vi "IsSearchGoalNode.vi"(8 "error in (no error)":errorcluster, 10 "PossibleSearchGoal in":refnum<data-value>, 11 "Tree in":refnum<class "Tree.lvclass">) -> (0 "error out":errorcluster, 1 "IsNode":bool, 2 "PossibleSearchGoal out":refnum<data-value>, 3 "Tree out":refnum<class "Tree.lvclass">)   [LabVIEW 2013, in "Tree.lvclass"]
doc: "Abstract method. Override this VI to implement a search of a tree. This VI is responsible for determining when we have found the node we are searching for."
uses:
  Tree.lvclass
  TreeNode/TreeNode.lvclass
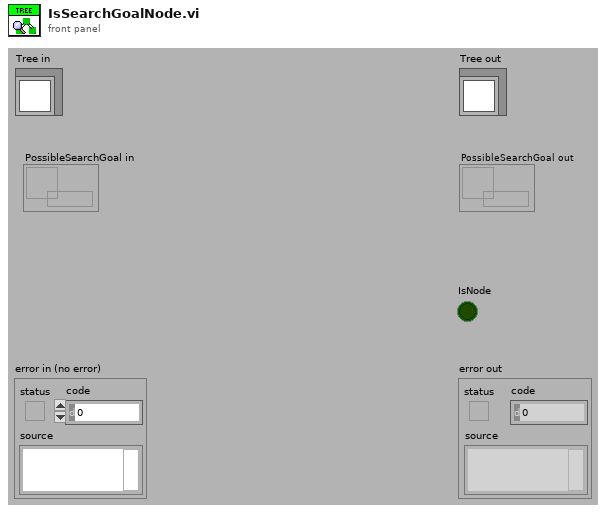
[diagram p1: front panel]
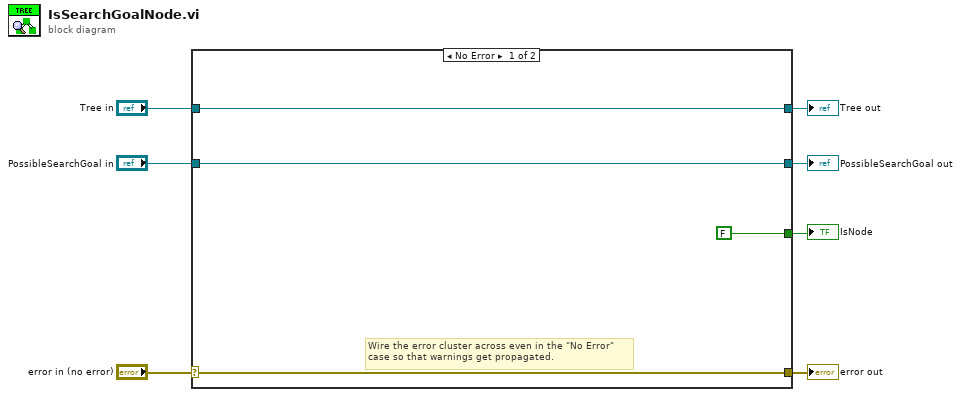
[diagram p0: block diagram]
diagram:
  n1 = case shown="No Error" "error in (no error)" {
    selector: "error in (no error)" -> [w10 w14]
    tunnel: [w10 w14] -> w6
    tunnel: [w11 w13] -> w4
    tunnel: "Tree in" -> [w11 w13]
    tunnel: "PossibleSearchGoal in" -> [w9 w12]
    tunnel: [w9 w12] -> w2
    tunnel: [FALSE _] -> w1
    frame No Error {
      # "Wire the error cluster across even in the \"No Error\"\ncase so that warnings get propagated."
    }
    frame Error {
    }
  }
  "error out" <- w6
  "Tree out" <- w4
  "PossibleSearchGoal out" <- w2
  "IsNode" <- w1
